vi "DAQ Control Standalone.vi"(5 "Serial Configuration":T2={"Baud Rate"=9600, "Parity"=0, "Data Bits"=8, "Stop Bits"=10, "Flow Control"=0} {"Flow Control" items=["None", "XON/XOFF", "RTS/CTS", "XON/XOFF & RTS/CTS", "DTR/DSR", "XON/XOFF & DTR/DSR"]; "Stop Bits" items=["1.0"=10, "1.5"=15, "2.0"=20]; "Data Bits" items=["7"=7, "8"=8]; "Parity" items=["None", "Odd", "Even", "Mark", "Space"]; "Baud Rate" items=["300"=300, "600"=600, "1200"=1200, "2400"=2400, "4800"=4800, "9600"=9600, "19200"=19200]}, 6 "Throttle":dbl, 7 "Serial Port Configuration":T3={"baud rate (9600)"=9600, "data bits (8)"=8, "parity (0:none)"=enum."None"} {"data bits (8)" min=5 max=8 step=1}, 8 "?":bool, 9 "PSU VISA":refnum<visa-resource-name>, 10 "DAQ Device Name":tag="cDAQ1Mod1", 11 "Fuelflow VISA":refnum<visa-resource-name>) -> (0 "Error Out":errorcluster, 1 "Power Supply Output":dbl[](array[numeric]), 2 "Power Output":cluster{"RPM":dbl, "Torque":dbl, "HP":dbl}, 3 "Fuelflow Output":T1, 4 "Mode":bool)   [LabVIEW 2014]
uses:
  <vilib>/Instr/_visa.llb/VISA Configure Serial Port (Instr).vi
  <vilib>/Utility/file.llb/Write To Spreadsheet File (string).vi
  <vilib>/DAQmx/read.llb/DAQmx Read (Analog 1D DBL NChan 1Samp).vi
  <vilib>/Utility/file.llb/Write To Spreadsheet File (DBL).vi
  <instrlib>/GPD-3303/GPD-3303.lvlib
panel:
  in  "Channel (1: Channel 1)":enum16{"Channel 1", "Channel 2"}(ring)=enum."Channel 2"
  out "Power supply Error Out":errorcluster
  out "Fuelflow Error Out":errorcluster
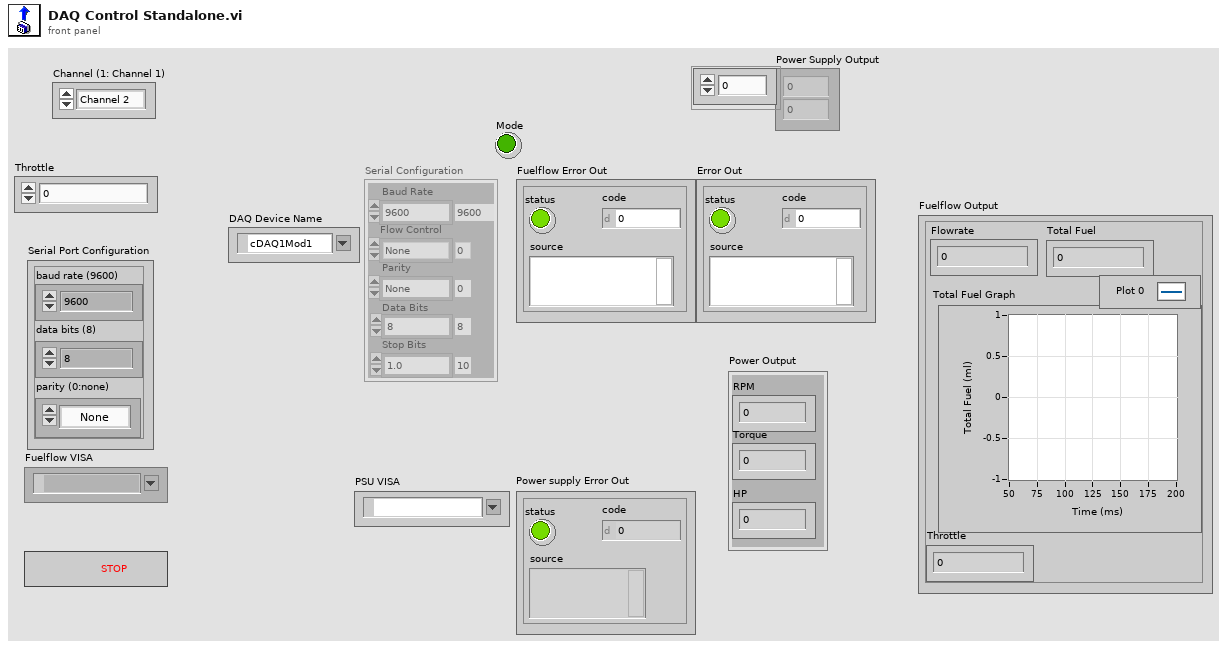
[diagram p1: front panel]
types:
  T1 = cluster{"Flowrate":dbl, "Total Fuel":dbl, "Total Fuel Graph":cluster{u32, dbl}[], "Throttle":dbl}
  T2 = cluster{"Baud Rate":u32, "Parity":u16, "Data Bits":u16, "Stop Bits":u16, "Flow Control":u16}
  T3 = cluster{"baud rate (9600)":u32, "data bits (8)":u16, "parity (0:none)":enum16{"None", "Odd", "Even", "Mark", "Space"}}
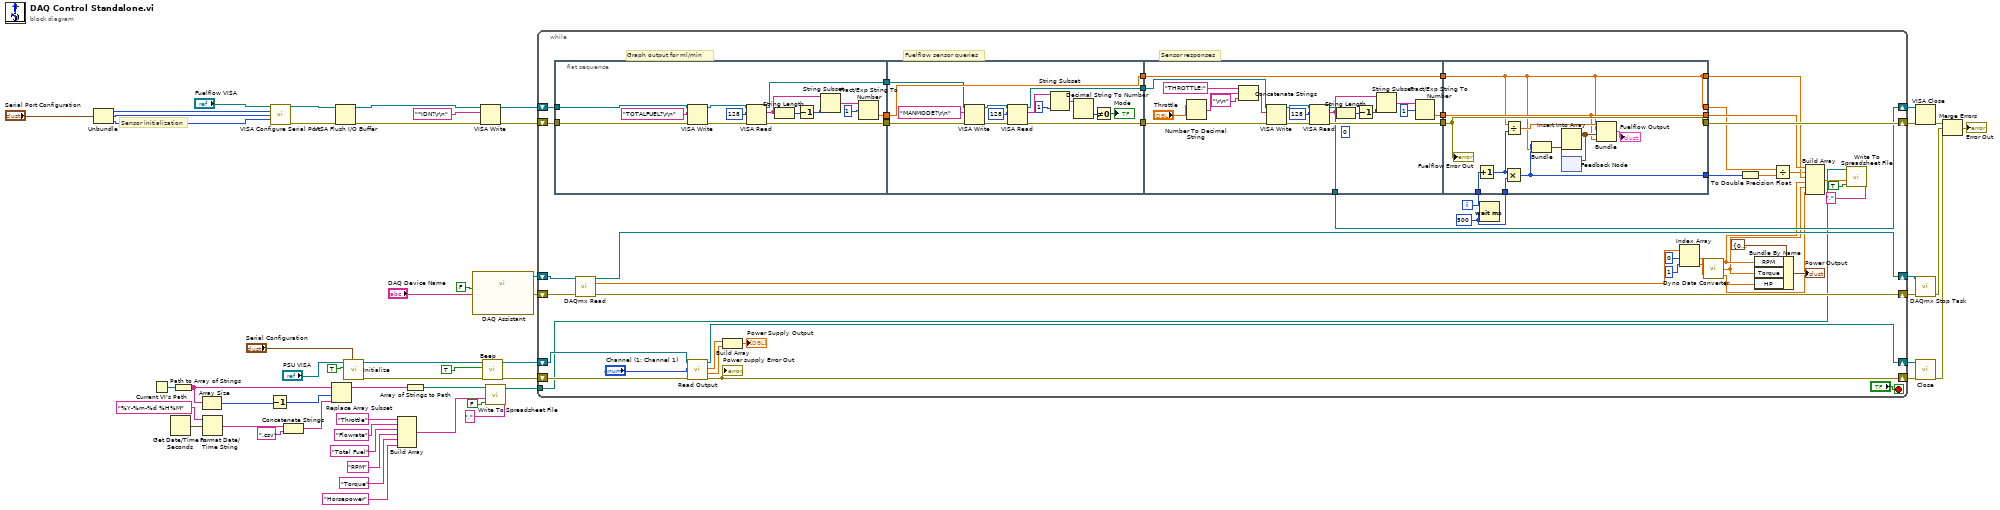
[diagram p0: block diagram]
diagram:
  # "Sensor initialization"
  n1 = Unbundle("Serial Port Configuration") -> ("baud rate (9600)"=w26:u32, "data bits (8)"=w25:u16, "parity (0:none)"=w24:enum16{"None", "Odd", "Even", "Mark", "Space"})
  n2 = Current VI's Path() -> (path=w6:path)
  n3 = Get Date/Time In Seconds() -> (seconds since 1Jan1904=w21:timestamp)
  n4 = Path to Array of Strings(0:w6) -> (2:w4:string[])  [unwired: 1 out]
  n5 = Array Size(array=w4) -> (size(s)=w3:i32)
  n6 = Format Date/Time String(time format string (%c)="%Y-%m-%d %H%M", seconds (now)=w21) -> (date/time string=w19:string)  [unwired: 1 in]
  n7 = Decrement(x=w3) -> (x-1=w2:i32)
  n8 = call-poly "VISA Configure Serial Port"("VISA resource name"="Fuelflow VISA", "baud rate (9600)"=w26, "data bits (8)"=w25, "parity (0:none)"=w24) -> ("VISA resource name out"=w29:refnum<visa-resource-name>, "error out"=w30:errorcluster)  [unwired: 10 in]
  n9 = Concatenate Strings(w19, ".csv" ("string")) -> (w5:string)
  n10 = Replace Array Subset(array=w4, new element=w5, index=w2) -> (w1:string[])
  n11 = VISA Flush I/O Buffer(VISA resource name=w29, error in (no error)=w30) -> (VISA resource name out=w27:refnum<visa-resource-name>, error out=w28:errorcluster)  [unwired: 1 in]
  n12 = call <instrlib>:"Initialize.vi"("Serial Configuration"="Serial Configuration", "ID Query (True)"=TRUE, "VISA resource name"="PSU VISA") -> ("error out"=w34:errorcluster, "VISA resource name out"=w35:refnum<visa-resource-name>)  [unwired: 7 in]
  n13 = Build Array("Throttle", "Flowrate" ("element"), "Total Fuel" ("element"), "RPM" ("element"), "Torque" ("element"), "Horsepower" ("element")) -> (w10:string[])
  n14 = Array of Strings to Path(0:w1) -> (2:w17:path)  [unwired: 1 in]
  n15 = call "DAQ Assistant"("stop (T)"=FALSE, "device name"="DAQ Device Name") -> ("task out"=w37:refnum<k21>, "error out"=w36:errorcluster)  [unwired: 15 in, 1 out]
  n16 = VISA Write(VISA resource name=w27, write buffer="*IDN?\r\n", error in (no error)=w28) -> (VISA resource name out=w22:refnum<visa-resource-name>, error out=w23:errorcluster)  [unwired: 1 out]
  n17 = call <instrlib>:"Beep.vi"("error in (no error)"=w34, "Enable Beep (T: Enable)"=TRUE, "VISA resource name"=w35) -> ("error out"=w47:errorcluster, "VISA resource name out"=w46:refnum<visa-resource-name>)  [unwired: 7 in]
  n18 = call-poly <vilib>:"Write To Spreadsheet File.vi"("delimiter (\\t)"="," ("delimiter (\\t)"), "append to file? (new file:F)"=FALSE, "1D data"=w10, "file path (dialog if empty)"=w17) -> ("new file path (Not A Path if cancelled)"=w7:path)  [unwired: 4 in]
  n19 = while {
    shift-right: [w82] -> w55
    shift-left: w22 -> [w83]
    shift-right: [w84] -> w54
    shift-left: w23 -> [w86]
    shift-right: [w102] -> w53
    shift-left: w46 -> [w103]
    shift-right: [w100] -> w52
    shift-left: w47 -> [w101]
    shift-right: [w96] -> w40
    shift-left: w37 -> [w97]
    shift-right: [w95] -> w39
    shift-left: w36 -> [w98]
    tunnel: w7 -> [w68]
    i -> [w89]
    stop <- "?" stop-if-true
    w81 = u32 500 ("milliseconds to wait")
    # "Graph output for ml/min"
    # "Sensor responses"
    # "Fuelflow sensor queries"
    n20 = flat-sequence {
      tunnel: [w115] -> w77
      tunnel: [w114] -> w75
      tunnel: w83 -> [w116]
      tunnel: w86 -> [w117]
      tunnel: [w113] -> w73
      tunnel: w77 -> [w130]
      tunnel: [w129] -> w76
      tunnel: w75 -> [w120]
      tunnel: [w118] -> w74
      tunnel: w73 -> [w131]
      tunnel: [w131] -> w72
      tunnel: w76 -> [w150]
      tunnel: w74 -> [w149]
      tunnel: [w148] -> w88
      tunnel: [w147] -> w87
      tunnel: [w146] -> w85
      tunnel: [w145] -> w82
      tunnel: w72 -> [w147]
      tunnel: w89 -> [w156]
      tunnel: w88 -> [w153]
      tunnel: w87 -> [w152]
      tunnel: w85 -> [w159]
      tunnel: [w159] -> w84
      tunnel: w81 -> [w154]
      tunnel: [w153] -> w65
      tunnel: [w152] -> w64
      tunnel: [w152] -> w59
      tunnel: [w151] -> w58
      frame #0 {
        n21 = VISA Write(VISA resource name=w116, write buffer="TOTALFUEL?\r\n", error in (no error)=w117) -> (VISA resource name out=w109:refnum<visa-resource-name>, error out=w110:errorcluster)  [unwired: 1 out]
        n22 = VISA Read(VISA resource name=w109, byte count=128, error in (no error)=w110) -> (VISA resource name out=w115:refnum<visa-resource-name>, read buffer=w104:string, error out=w114:errorcluster)  [unwired: 1 out]
        n23 = String Length(string=w104) -> (length=w107:i32)
        n24 = Decrement(x=w107) -> (x-1=w106:i32)
        n25 = String Subset(string=w104, length (rest)=w106) -> (substring=w105:string)  [unwired: 1 in]
        n26 = Fract/Exp String To Number(string=w105, offset=1) -> (number=w113:dbl)  [unwired: 2 in, 1 out]
      }
      frame #1 {
        n27 = VISA Write(VISA resource name=w130, write buffer="MANMODE?\r\n", error in (no error)=w120) -> (VISA resource name out=w126:refnum<visa-resource-name>, error out=w119:errorcluster)  [unwired: 1 out]
        n28 = VISA Read(VISA resource name=w126, byte count=u32 128, error in (no error)=w119) -> (VISA resource name out=w129:refnum<visa-resource-name>, read buffer=w123:string, error out=w118:errorcluster)  [unwired: 1 out]
        n29 = String Subset(string=w123, length (rest)=1 ("length (rest)")) -> (substring=w121:string)  [unwired: 1 in]
        n30 = Decimal String To Number(string=w121) -> (number=w128:i32)  [unwired: 2 in, 1 out]
        n31 = Not Equal To 0?(x=w128) -> (x != 0?=→"Mode":bool)
      }
      frame #2 {
        (unwired) i16 0 ("width (-)")
        n32 = Number To Decimal String(number="Throttle") -> (decimal integer string=w139:string)  [unwired: 1 in]
        n33 = Concatenate Strings("THROTTLE:" ("string"), w139, "\r\n" ("string")) -> (w137:string)
        n34 = VISA Write(VISA resource name=w150, write buffer=w137, error in (no error)=w149) -> (VISA resource name out=w143:refnum<visa-resource-name>, error out=w142:errorcluster)  [unwired: 1 out]
        n35 = VISA Read(VISA resource name=w143, byte count=128, error in (no error)=w142) -> (VISA resource name out=w145:refnum<visa-resource-name>, read buffer=w133:string, error out=w146:errorcluster)  [unwired: 1 out]
        n36 = String Length(string=w133) -> (length=w135:i32)
        n37 = Decrement(x=w135) -> (x-1=w134:i32)
        n38 = String Subset(string=w133, length (rest)=w134) -> (substring=w136:string)  [unwired: 1 in]
        n39 = Fract/Exp String To Number(string=w136, offset=1) -> (number=w148:dbl)  [unwired: 2 in, 1 out]
      }
      frame #3 {
        n40 = Increment(x=w156) -> (x+1=w155:i32)
        n41 = Multiply(x=w155, y=w154) -> (x*y=w151:u32)
        n42 = Divide(x=w152, y=w155) -> (x/y=w158:dbl)
        n43 = Bundle(w151, w152) -> (w162:cluster{u32, dbl})  [unwired: 1 in]
        n44 = feedback #1() -> (w161:cluster{u32, dbl}[])  [unwired: 1 in]
        n45 = Insert Into Array(array=w161, new element=w162) -> (w160:cluster{u32, dbl}[])  [unwired: 1 in]
        n46 = feedback-in #1(w160) -> ()
        n47 = Bundle(w158, w152, w160, w153) -> (→"Fuelflow Output":cluster{dbl, dbl, cluster{u32, dbl}[], dbl})  [unwired: 1 in]
        "Fuelflow Error Out" <- w159
      }
    }
    n48 = call-poly <vilib>:"DAQmx Read.vi"("task/channels in"=w97, "error in"=w98) -> ("task out"=w96:refnum<k21>, "data"=w94:dbl[], "error out"=w95:errorcluster)  [unwired: 11 in]
    n49 = call <instrlib>:"Read Output.vi"("error in (no error)"=w101, "Channel (1: Channel 1)"="Channel (1: Channel 1)", "VISA resource name"=w103) -> ("error out"=w100:errorcluster, "Actual Current Level (A)"=w79:dbl, "Actual Voltage Level (V)"=w80:dbl, "VISA resource name out"=w102:refnum<visa-resource-name>)  [unwired: 5 in]
    "Power supply Error Out" <- w100
    n50 = Build Array(w80, w79) -> (→"Power Supply Output":dbl[])
    n51 = Wait (ms)(milliseconds to wait=w81) -> ()  [unwired: 1 out]
    n52 = Index Array(array=w94, index #1=0 ("index"), index #2=1 ("index")) -> (element #1=w91:dbl, element #2=w90:dbl)
    n53 = call "Dyno Data Converter.vi"("VShunt"=w90, "VGen"=w91) -> ("RPM"=w63:dbl, "Torque"=w62:dbl, "HP"=w61:dbl)
    n54 = To Double Precision Float(number=w58) -> (double precision float=w56:dbl)
    n55 = Bundle By Name(cluster=cluster{"RPM":dbl, "Torque":dbl, "HP":dbl} {"RPM"=0.0, "Torque"=0.0, "HP"=0.0} ("Power Output"), "RPM"=w63, "Torque"=w62, "HP"=w61) -> (→"Power Output":cluster{"RPM":dbl, "Torque":dbl, "HP":dbl})
    n56 = Divide(x=w59, y=w56) -> (x/y=w57:dbl)
    n57 = Build Array(w65, w57, w64, w63, w62, w61) -> (w66:dbl[])
    n58 = call-poly <vilib>:"Write To Spreadsheet File.vi"("delimiter (\\t)"="," ("delimiter (\\t)"), "append to file? (new file:F)"=TRUE, "1D data"=w66, "file path (dialog if empty)"=w68) -> ()  [unwired: 4 in, 1 out]
  }
  n59 = VISA Close(VISA resource name=w55, error in (no error)=w54) -> (error out=w51:errorcluster)
  n60 = call <vilib>:"DAQmx Stop Task.vi"("task/channels in"=w40, "error in"=w39) -> ("error out"=w41:errorcluster)  [unwired: 12 in, 1 out]
  n61 = call <instrlib>:"Close.vi"("error in (no error)"=w52, "VISA resource name"=w53) -> ("error out"=w42:errorcluster)  [unwired: 9 in]
  n62 = Merge Errors(w51, w41, w42) -> (→"Error Out":errorcluster)
